vi "Coord window-Generate rectangle coordinates.vi"(9 "Normalised Effective FOV/2":T1, 11 "Norm point(x,y) (for display)":cluster{"x":i16, "y":i16}) -> (3 "Norm rect (for display)":T2)   [LabVIEW 2013]
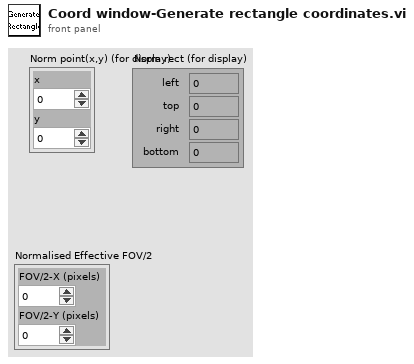
[diagram p1: front panel]
types:
  T1 = cluster{"FOV/2-X (pixels)":i16, "FOV/2-Y (pixels)":i16}
  T2 = cluster{"left":i16, "top":i16, "right":i16, "bottom":i16}
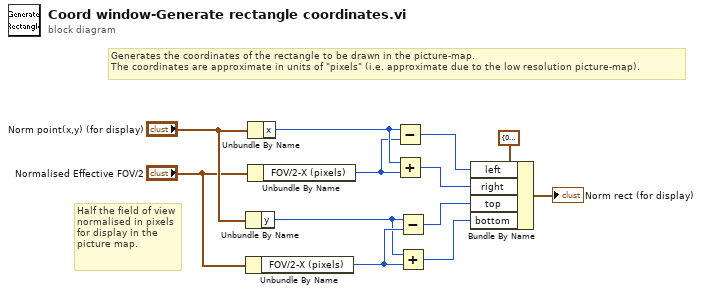
[diagram p0: block diagram]
diagram:
  # "Generates the coordinates of the rectangle to be drawn in the picture-map.\nThe coordinates are approximate in units of \"pixels\" (i.e. approximate due to the low resolution picture-map)."
  # "Half the field of view normalised in pixels for display in the picture map."
  n1 = Unbundle By Name("Norm point(x,y) (for display)") -> ("y"=w4:i16)
  n2 = Unbundle By Name("Normalised Effective FOV/2") -> ("FOV/2-X (pixels)"=w5:i16)
  n3 = Unbundle By Name("Norm point(x,y) (for display)") -> ("x"=w8:i16)
  n4 = Unbundle By Name("Normalised Effective FOV/2") -> ("FOV/2-X (pixels)"=w7:i16)
  n5 = Subtract(x=w8, y=w7) -> (x-y=w9:i16)
  n6 = Add(x=w8, y=w7) -> (x+y=w6:i16)
  n7 = Subtract(x=w4, y=w5) -> (x-y=w3:i16)
  n8 = Add(x=w4, y=w5) -> (x+y=w1:i16)
  n9 = Bundle By Name(cluster=T2 {"left"=0, "top"=0, "right"=0, "bottom"=0} ("Norm rect (for display)"), "left"=w9, "right"=w6, "top"=w3, "bottom"=w1) -> (→"Norm rect (for display)":T2)
